vi "SPR_01.vi"(2 "select":T1(ring), 5 "key":string, 11 "error in":errorcluster) -> (4 "Certificate":u8, 6 "found":bool, 15 "error out":errorcluster)   [LabVIEW 2011]
uses:
  <vilib>/Utility/file.llb/Write To Spreadsheet File (string).vi
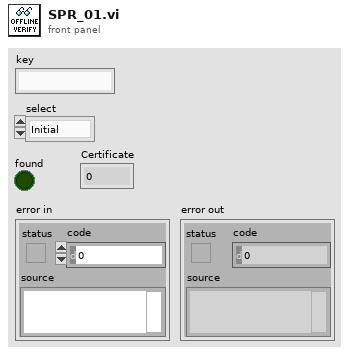
[diagram p1: front panel]
types:
  T1 = enum16{"Initial", "Insert", "Delete", "Search", "Release"}
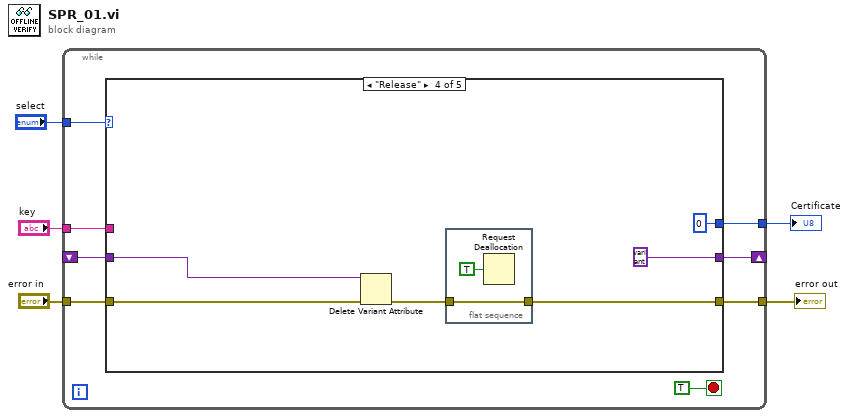
[diagram p0: block diagram]
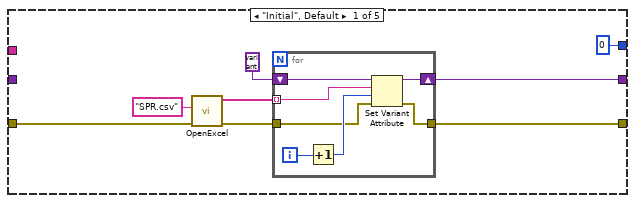
[diagram p2: hidden frame]
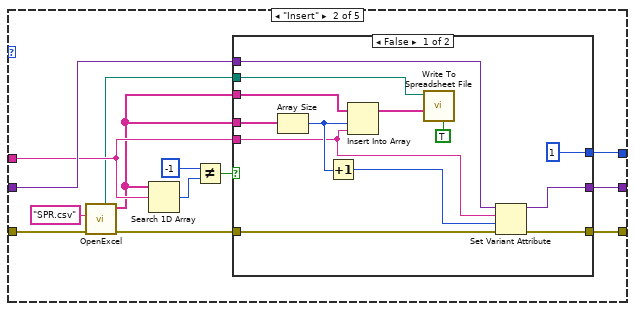
[diagram p3: hidden frame]
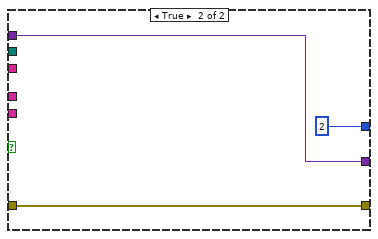
[diagram p4: hidden frame]
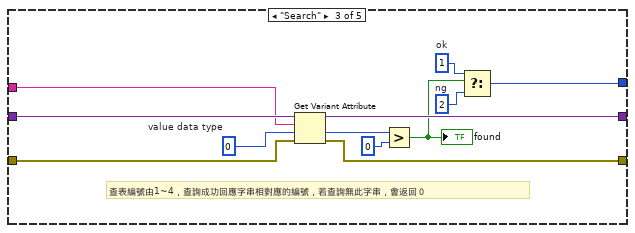
[diagram p5: hidden frame]
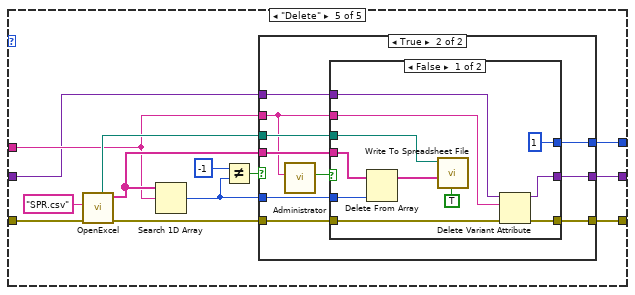
[diagram p6: hidden frame]
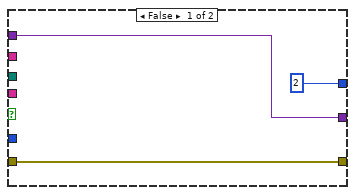
[diagram p7: hidden frame]
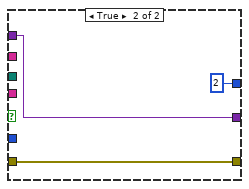
[diagram p8: hidden frame]
diagram:
  n1 = while {
    shift-right: [w13] -> _
    shift-left: _ -> [w12]
    tunnel: "key" -> [w10]
    tunnel: "select" -> [w9]
    tunnel: [w8] -> w3
    tunnel: "error in" -> [w7]
    tunnel: [w6] -> w2
    stop <- TRUE stop-if-true
    n2 = case shown="\"Release\"" w9 {
      tunnel: [w20 w39 w67 variant ("variant") w79] -> w13
      tunnel: w12 -> [_ w40 w68 w75 w80]
      tunnel: w10 -> [_ w33 w64 _ w81]
      tunnel: [w19 w41 w62 w71 w83] -> w8
      tunnel: w7 -> [w17 w38 w63 w73 w90]
      tunnel: [u8 0 w30 w58 u8 0 w82] -> w6
      frame "Initial", Default {
        n3 = call "OpenExcel.vi"("error in (no error)"=w17, "name or relative path"="SPR.csv") -> ("error out"=w16:errorcluster, "all rows"=w18:string[])  [unwired: 7 in, 1 out]
        n4 = for {
          shift-right: [w27] -> w20
          shift-left: variant ("variant") -> [w28]
          tunnel: w18 -> [w26] mode=indexing
          tunnel: w16 -> [w23]
          tunnel: [w22] -> w19
          i -> [w24]
          n5 = Increment(x=w24) -> (x+1=w25:i32)
          n6 = Set Variant Attribute(Variant=w28, name=w26, value=w25, error in=w23) -> (Variant out=w27:variant, error out=w22:errorcluster)  [unwired: 1 out]
        }
      }
      frame "Insert" {
        n7 = call "OpenExcel.vi"("error in (no error)"=w38, "name or relative path"="SPR.csv") -> ("error out"=w34:errorcluster, "all rows"=w32:string[], "appended path"=w31:path)  [unwired: 7 in]
        n8 = Search 1D Array(1D array=w32, element=w33) -> (index of element=w37:i32)  [unwired: 1 in]
        n9 = Not Equal?(x=-1, y=w37) -> (x != y?=w35:bool)
        n10 = case shown="False" w35 {
          tunnel: [w53 w57] -> w41
          tunnel: w40 -> [w54 w56]
          tunnel: [w52 w56] -> w39
          tunnel: w32 -> [w51 _]
          tunnel: w34 -> [w43 w57]
          tunnel: w33 -> [w47 _]
          tunnel: w32 -> [w50 _]
          tunnel: w31 -> [w46 _]
          tunnel: [u8 1 u8 2] -> w30
          frame False {
            n11 = Array Size(array=w51) -> (size(s)=w49:i32)
            n12 = Increment(x=w49) -> (x+1=w48:i32)
            n13 = Insert Into Array(array=w50, index=w49, new element=w47) -> (w44:string[])
            n14 = call-poly <vilib>:"Write To Spreadsheet File.vi"("transpose? (no:F)"=TRUE, "1D data"=w44, "file path (dialog if empty)"=w46) -> ()  [unwired: 5 in, 1 out]
            n15 = Set Variant Attribute(Variant=w54, name=w47, value=w48, error in=w43) -> (Variant out=w52:variant, error out=w53:errorcluster)  [unwired: 1 out]
          }
          frame True {
          }
        }
      }
      frame "Search" {
        w60 = u8 2  # ng
        w59 = u8 1  # ok
        w69 = 0  # value data type
        # "查表編號由1~4，查詢成功回應字串相對應的編號，若查詢無此字串，會返回０"
        n16 = Get Variant Attribute(Variant=w68, name=w64, default value (empty Variant)=w69, error in=w63) -> (duplicate Variant=w67:variant, value=w66:i32, error out=w62:errorcluster)  [unwired: 1 out]
        n17 = Greater?(x=w66, y=0) -> (0:w61:bool)
        "found" <- w61
        n18 = Select(t=w59, s=w61, f=w60) -> (s? t:f=w58:u8)
      }
      frame "Release" {
        n19 = Delete Variant Attribute(4:w73, 7:w75) -> (0:w72:errorcluster)  [unwired: 1 in, 2 out]
        n20 = flat-sequence {
          tunnel: w72 -> [w76]
          tunnel: [w76] -> w71
          frame #0 {
            n21 = Request Deallocation(TRUE ("flag")) -> ()
          }
        }
      }
      frame "Delete" {
        n22 = call "OpenExcel.vi"("error in (no error)"=w90, "name or relative path"="SPR.csv") -> ("error out"=w85:errorcluster, "all rows"=w86:string[], "appended path"=w84:path)  [unwired: 7 in]
        n23 = Search 1D Array(1D array=w86, element=w81) -> (index of element=w88:i32)  [unwired: 1 in]
        n24 = Not Equal?(x=-1, y=w88) -> (x != y?=w87:bool)
        n25 = case shown="True" w87 {
          tunnel: w88 -> [_ w103]
          tunnel: w86 -> [_ w102]
          tunnel: w85 -> [w93 w100]
          tunnel: w84 -> [_ w101]
          tunnel: [w93 w99] -> w83
          tunnel: [u8 2 w94] -> w82
          tunnel: w81 -> [_ w96]
          tunnel: w80 -> [w91 w98]
          tunnel: [w91 w97] -> w79
          frame False {
          }
          frame True {
            n26 = call "Administrator.vi"("string"=w96) -> ("on/off"=w95:bool)  [unwired: 10 in]
            n27 = case shown="False" w95 {
              tunnel: w103 -> [w114 _]
              tunnel: w102 -> [w113 _]
              tunnel: w101 -> [w111 _]
              tunnel: w100 -> [w109 w116]
              tunnel: [w108 w116] -> w99
              tunnel: w98 -> [w107 w117]
              tunnel: [w106 w117] -> w97
              tunnel: w96 -> [w105 _]
              tunnel: [u8 1 u8 2] -> w94
              frame False {
                n28 = Delete From Array(array=w113, index=w114) -> (array with subset deleted=w112:string[])  [unwired: 1 in, 1 out]
                n29 = call-poly <vilib>:"Write To Spreadsheet File.vi"("transpose? (no:F)"=TRUE, "1D data"=w112, "file path (dialog if empty)"=w111) -> ()  [unwired: 5 in, 1 out]
                n30 = Delete Variant Attribute(4:w109, 6:w105, 7:w107) -> (0:w108:errorcluster, 3:w106:variant)  [unwired: 1 out]
              }
              frame True {
              }
            }
          }
        }
      }
    }
  }
  "error out" <- w3
  "Certificate" <- w2
